vi "RSZVB Get Mixer Delay Constant.vi"(8 "error in (no error)":errorcluster {"code" format="%.0x"}, 10 "Channel (1)":i32=1, 11 "VISA session":refnum<visa-resource-name>) -> (0 "error out":errorcluster {"code" format="%.0x"}, 1 "Constant Delay":dbl format="%^.3e", 3 "dup VISA session":refnum<visa-resource-name>)   [LabVIEW 2011]
doc: "Returns a constant mixer delay value, to be used as a reference for a mixer delay measurement calibration.\n\nRemote-control command(s):\n[SENSe<Ch>:]FREQuency:MDELay:CDELay?"
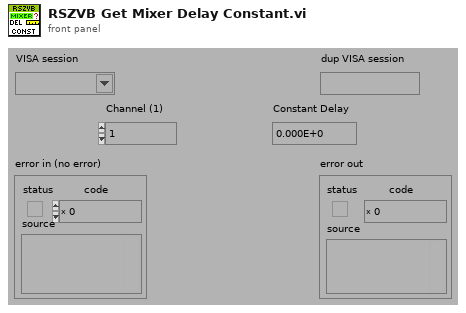
[diagram p1: front panel]
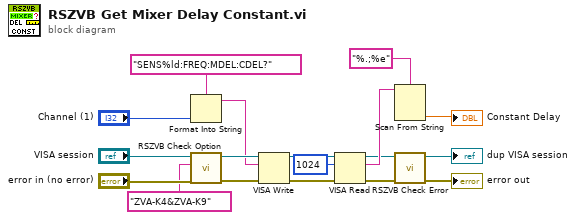
[diagram p0: block diagram]
diagram:
  n1 = Format Into String(format string="SENS%ld:FREQ:MDEL:CDEL?", "Channel (1)") -> (resulting string=w11:string)  [unwired: 2 in, 1 out]
  n2 = call "RSZVB Check Option.vi"("error in (no error)"="error in (no error)", "Options"="ZVA-K4&ZVA-K9", "VISA session"="VISA session") -> ("error out"=w13:errorcluster, "dup VISA session"=w12:refnum<visa-resource-name>)  [unwired: 7 in]
  n3 = VISA Write(VISA resource name=w12, write buffer=w11, error in (no error)=w13) -> (VISA resource name out=w9:refnum<visa-resource-name>, error out=w10:errorcluster)  [unwired: 1 out]
  n4 = VISA Read(VISA resource name=w9, byte count=u32 1024, error in (no error)=w10) -> (VISA resource name out=w3:refnum<visa-resource-name>, read buffer=w7:string, error out=w6:errorcluster)  [unwired: 1 out]
  n5 = Scan From String(format string="%.;%e", input string=w7) -> (output 1=→"Constant Delay":dbl)  [unwired: 3 in, 3 out]
  n6 = call "RSZVB Check Error.vi"("error in (no error)"=w6, "VISA session"=w3) -> ("error out"=→"error out":errorcluster, "dup VISA session"=→"dup VISA session":refnum<visa-resource-name>)  [unwired: 8 in]
